vi "Memory.Pointer.Copy All.Safe.vi"(8 "error in (no error)":errorcluster, 10 "dst pointer in":refnum<class "Memory.Pointer.lvclass">, 11 "src pointer in":refnum<class "Memory.Pointer.lvclass">) -> (0 "error out":errorcluster, 2 "dst pointer out":refnum<class "Memory.Pointer.lvclass">, 3 "src pointer out":refnum<class "Memory.Pointer.lvclass">)   [LabVIEW 2016, in "Memory Manager.lvlib" / "Memory.Pointer.lvclass"]
doc: "Copies all of the data stored at the memory location of the <b>src pointer</b> into the memory address associated with <b>dst pointer</b>.\n\n<b>Note:</b> This VI is <b>safe</b>.\n\nSafe means that this function evaluates that the size parameter of <b>dst pointer</b> is greater than or equal to the size of <b>src pointer</b> to ensure that the destination memory location is an appropriate size before copying data from source to destination. Reading/writing more data to a pointer than it has allocated can corrupt or crash LabVIEW."
uses:
  Memory.Pointer.lvclass
  Memory.Pointer.lvclass/Memory.Pointer.ctl
  Memory.Pointer.Copy.Unsafe.vi
  Accessors/Get Address.vi
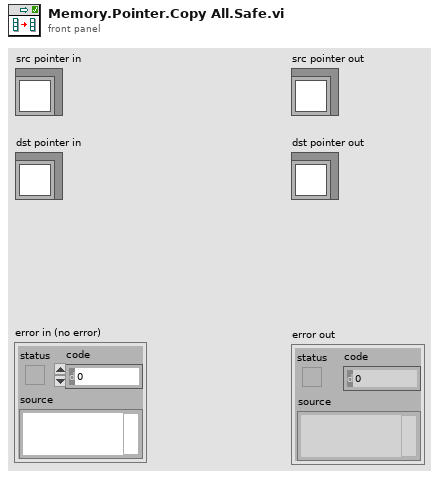
[diagram p1: front panel]
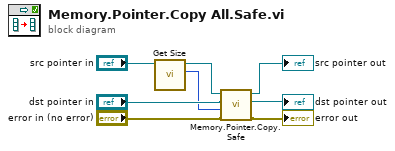
[diagram p0: block diagram]
diagram:
  n1 = call "Get Size.vi"("Pointer in"="src pointer in") -> ("size"=w5:u64, "Pointer out"=w7:refnum<class "Memory.Pointer.lvclass">)  [unwired: 8 in, 1 out]
  n2 = call "Memory.Pointer.Copy.Safe.vi"("error in (no error)"="error in (no error)", "bytes to copy"=w5, "dst pointer in"="dst pointer in", "src pointer in"=w7) -> ("error out"=→"error out":errorcluster, "dst pointer out"=→"dst pointer out":refnum<class "Memory.Pointer.lvclass">, "src pointer out"=→"src pointer out":refnum<class "Memory.Pointer.lvclass">)  [unwired: 4 in, 1 out]
